vi "Buttons and Lights.vi"() -> ()   [LabVIEW 2011]
panel:
  in  "Power Meter":dbl(slide) scale=0.0..10.0
  out "Measured Power":dbl
  out "Kill":bool
  in  "Safety":bool
  out "Safety Indic":bool
  in  "stop":bool
  in  "Door Open":bool
  out "Door Open Indic":bool
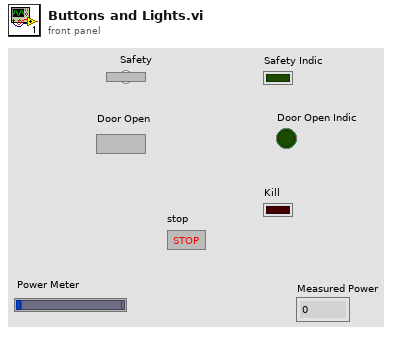
[diagram p1: front panel]
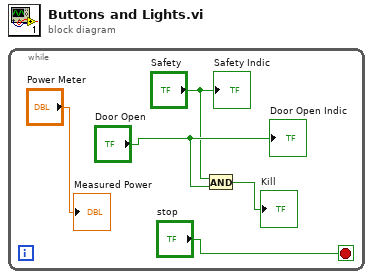
[diagram p0: block diagram]
diagram:
  n1 = while {
    stop <- "stop" stop-if-true
    n2 = And(x="Safety", y="Door Open") -> (x .and. y?=→"Kill":bool)
    "Door Open Indic" <- "Door Open"
    "Safety Indic" <- "Safety"
    "Measured Power" <- "Power Meter"
  }
